vi "Mobility-Vt-Used Pts_Saturation_09_11_12a_JW.vi"(5 "Width":dbl, 7 "Length":dbl, 9 "Dielectric (d)":dbl, 10 "Sat Id Used":dbl[](array[numeric]), 11 "Vg Used":dbl[](array[numeric])) -> (1 "Capacitance":dbl, 2 "Vt":dbl, 3 "Mobility":dbl)   [LabVIEW 2011]
uses:
  <vilib>/Analysis/NI_AALPro.lvlib
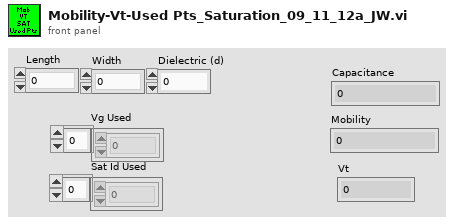
[diagram p1: front panel]
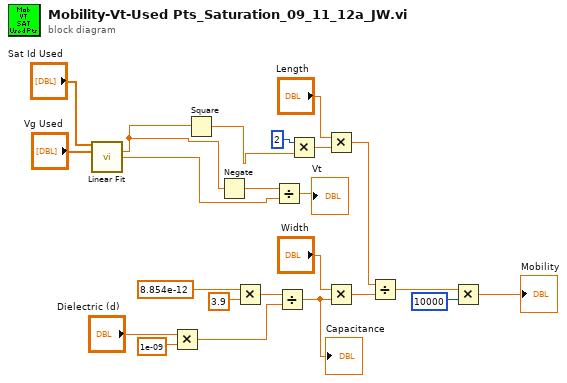
[diagram p0: block diagram]
diagram:
  n1 = call <vilib>:"Linear Fit.vi"("Y"="Sat Id Used", "X"="Vg Used") -> ("slope"=w1:dbl, "intercept"=w3:dbl)  [unwired: 9 in, 3 out]
  n2 = Multiply(x="Dielectric (d)", y=1e-09) -> (x*y=w22:dbl)
  n3 = Square(x=w1) -> (x^2=w2:dbl)
  n4 = Negate(x=w1) -> (-x=w5:dbl)
  n5 = Multiply(x=8.854e-12, y=3.9) -> (x*y=w23:dbl)
  n6 = Divide(x=w5, y=w3) -> (x/y=→"Vt":dbl)
  n7 = Divide(x=w23, y=w22) -> (x/y=w4:dbl)
  "Capacitance" <- w4
  n8 = Multiply(x=2, y=w2) -> (x*y=w15:dbl)
  n9 = Multiply(x="Length", y=w15) -> (x*y=w14:dbl)
  n10 = Multiply(x="Width", y=w4) -> (x*y=w13:dbl)
  n11 = Divide(x=w14, y=w13) -> (x/y=w11:dbl)
  n12 = Multiply(x=w11, y=10000) -> (x*y=→"Mobility":dbl)
